vi "Check Message.vi"(2 "Message":string, 3 "Expression":string) -> (1 "Correct Message":bool)   [LabVIEW 2023]
uses:
  <vilib>/regexp/Match Regular Expression.xnode
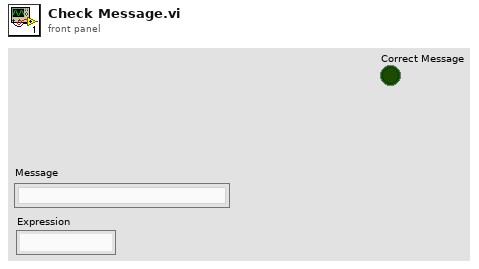
[diagram p1: front panel]
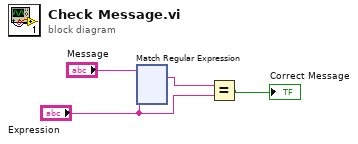
[diagram p0: block diagram]
diagram:
  n1 = xnode "Match Regular Expression"("input string"="Message", "regular expression"="Expression") -> ("whole match"=w3:string)  [unwired: 4 in, 4 out]
  n2 = Equal?(x=w3, y="Expression") -> (x = y?=→"Correct Message":bool)
